vi "Create Cartesian Offsets.vi"(8 "error in (no error)":errorcluster, 10 "Tag":string, 11 "LBCB Number":T3) -> (0 "error out":errorcluster, 1 "Cart Force Offsets":T1, 3 "Cart Disp Offsets":T2)   [LabVIEW 2009]
uses:
  Data Access Objects/Metadata/LBCB Number.ctl
  Data Access Objects/Metadata/Cartesian Point.ctl
  Data Access Objects/Metadata/Cartesian Force Vector.ctl
  Data Access Objects/Metadata/DAO Actions.ctl
  Data Access Objects/Metadata/Persistant DAO Actions.ctl
  Control Loop/LBCB_Conversions_Actions.ctl
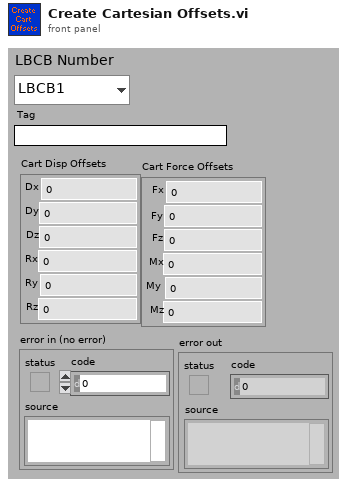
[diagram p1: front panel]
types:
  T1 = typedef "Cartesian Force Vector.ctl" = cluster{"Fx":dbl, "Fy":dbl, "Fz":dbl, "Mx":dbl, "My":dbl, "Mz":dbl}
  T2 = typedef "Cartesian Point.ctl" = cluster{"Dx":dbl, "Dy":dbl, "Dz":dbl, "Rx":dbl, "Ry":dbl, "Rz":dbl}
  T3 = typedef "LBCB Number.ctl" = enum16{"LBCB1", "LBCB2"}
  T4 = typedef "LBCB_Conversions_Actions.ctl" = enum16{"A2C", "C2A", "Set Log Filename", "Init"}
  T5 = typedef "Persistant DAO Actions.ctl" = enum16{"Init", "Get", "Set", "Load", "Save"}
  T6 = typedef "DAO Actions.ctl" = enum16{"Init", "Get", "Set"}
  T7 = typedef "LBCB Settings.ctl" = cluster{"Size":T8, "Type":T9}
  T8 = typedef "LBCB Size.ctl" = enum16{"1/5th-scale LBCB", "Full-scale LBCB", "Portable LBCB"}
  T9 = typedef "LBCB Type.ctl" = enum16{"X Actuators On The Left", "X Actuators On The Right"}
  T10 = typedef "LBCB Position.ctl" = cluster{"Motion Center":dbl[], "Transformation Matrix":dbl[][]}
  T11 = typedef "Actuator Point.ctl" = cluster{"X1":dbl, "X2":dbl, "Y1":dbl, "Z1":dbl, "Z2":dbl, "Z3":dbl}
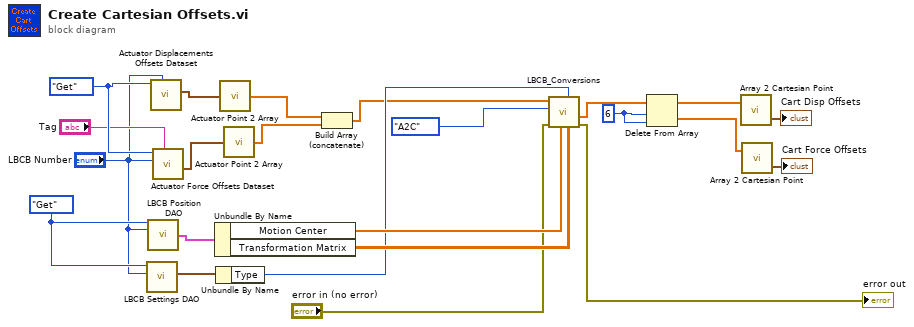
[diagram p0: block diagram]
diagram:
  w3 = 6 ("length")
  w16 = Persistant_DAO_Actions."Get" ("LBCB Settings Actions")
  w23 = DAO_Actions."Get" ("DAO Actions")
  n1 = call "LBCB Settings DAO.vi"("LBCB Number"="LBCB Number", "Actions"=w16) -> ("LBCB Setting Out"=w21:T7)  [unwired: 7 in, 2 out]
  n2 = call "LBCB Position DAO.vi"("LBCB Settings Actions"=w16, "LBCB Number"="LBCB Number") -> ("LBCB Position Output"=w20:T10)  [unwired: 11 in, 2 out]
  n3 = call "Actuator Displacements Offsets Dataset.vi"("LBCB Number"="LBCB Number", "DAO Actions"=w23) -> ("Offsets Out"=w9:T11)  [unwired: 8 in, 1 out]
  n4 = call "Actuator Force Offsets Dataset.vi"("Tag"="Tag", "LBCB Number"="LBCB Number", "DAO Actions"=w23) -> ("Offsets Out"=w8:T11)  [unwired: 6 in, 2 out]
  n5 = Unbundle By Name(w20) -> ("Motion Center"=w14:dbl[], "Transformation Matrix"=w13:dbl[][])
  n6 = Unbundle By Name(w21) -> ("Type"=w12:T9)
  n7 = call "Actuator Point 2 Array.vi"("Actuator Point"=w9) -> ("Array"=w7:dbl[])
  n8 = call "Actuator Point 2 Array.vi"("Actuator Point"=w8) -> ("Array"=w6:dbl[])
  n9 = Build Array (concatenate)(w7, w6) -> (w5:dbl[])
  n10 = call "LBCB_Conversions.vi"("Transformation Matrix"=w13, "Type"=w12, "Motion Center"=w14, "error in (no error)"="error in (no error)", "Conversion Type"=LBCB_Conversions_Actions."A2C", "Input"=w5) -> ("error out"=→"error out":errorcluster, "Output"=w18:dbl[])  [unwired: 4 in]
  n11 = Delete From Array(array=w18, length=w3, index=w3) -> (deleted portion=w2:dbl[], array with subset deleted=w4:dbl[])
  n12 = call "Array 2 Cartesian Point.vi"("Array"=w4) -> ("Cart Disp"=→"Cart Disp Offsets":T2)  [unwired: 2 in]
  n13 = call "Array 2 Cartesian Point.vi"("Array"=w2) -> ("Cart Disp"=→"Cart Force Offsets":T2)  [unwired: 2 in]
